vi "Get Missing Dependencies.vi"(8 "error in":errorcluster, 9 "shared directory":path, 10 "outside vis in":string[](array[string]), 11 "measurement directory":path) -> (0 "error out":errorcluster, 3 "outside vis out":string[](array[string]))   [LabVIEW 2021, in "Multiple Converter.lvlib"]
uses:
  Multiple Converter.lvlib
  e56e842d-5902-469a-bbd5-1077467e5c47.vi
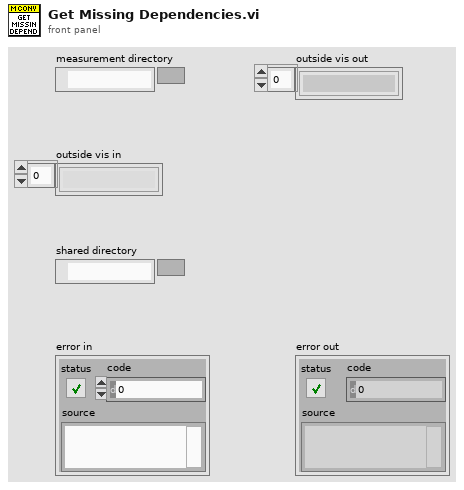
[diagram p1: front panel]
types:
  T1 = typedef "LVMissingDepInfoTypeDef.ctl" = cluster{"Missing Path":path, "Missing Name":string, "Missing Type":string}[]
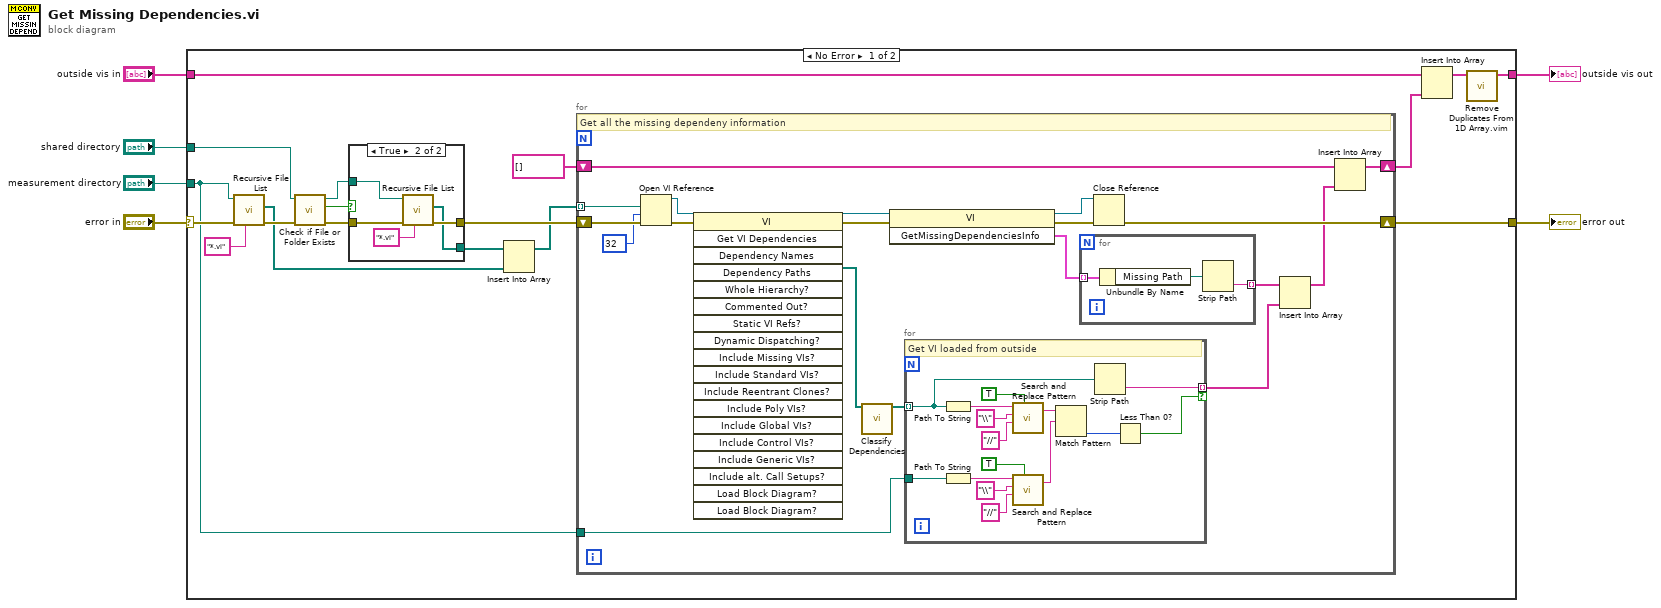
[diagram p0: block diagram]
diagram:
  n1 = case shown="No Error" "error in" {
    selector: "error in" -> [w24 w69]
    tunnel: [w21 w69] -> w5
    tunnel: "measurement directory" -> [w11 _]
    tunnel: "outside vis in" -> [w19 w68]
    tunnel: [w18 w68] -> w2
    tunnel: "shared directory" -> [w8 _]
    frame No Error {
      n2 = call <vilib>:"Recursive File List.vi"("pattern"="*.vi", "error in (no error)"=w24, "Folder Path"=w11) -> ("error out"=w16:errorcluster, "All Files in Dir"=w13:path[])  [unwired: 4 in, 3 out]
      n3 = call <vilib>:"Check if File or Folder Exists.vi"("error in (no error)"=w16, "path"=w8) -> ("error out"=w10:errorcluster, "file or folder exists?"=w9:bool, "dup path"=w7:path)  [unwired: 7 in]
      n4 = case shown="True" w9 {
        tunnel: w10 -> [w25 w29]
        tunnel: [w25 w28] -> w15
        tunnel: [_ w27] -> w14
        tunnel: w7 -> [_ w26]
        frame False {
        }
        frame True {
          n5 = call <vilib>:"Recursive File List.vi"("pattern"="*.vi", "error in (no error)"=w29, "Folder Path"=w26) -> ("error out"=w28:errorcluster, "All Files in Dir"=w27:path[])  [unwired: 4 in, 3 out]
        }
      }
      n6 = Insert Into Array(array=w14, new element=w13) -> (w12:path[])  [unwired: 1 in]
      n7 = for {
        tunnel: w12 -> [w49] mode=indexing
        shift-right: [w44] -> w21
        shift-left: w15 -> [w42]
        tunnel: w11 -> [w38]
        shift-right: [w35] -> w23
        shift-left: string[] [] -> [w36]
        # "Get all the missing dependeny information"
        n8 = Open VI Reference(vi path=w49, options=32, error in (no error)=w42) -> (vi reference=w40:refnum<vi>, error out=w48:errorcluster)  [unwired: 3 in]
        n9 = invoke class="VI" method="Get VI Dependencies"(reference=w40, error in=w48) -> (reference out=w39:refnum<vi>, error out=w41:errorcluster, "Dependency Paths"=w33:path[])  [unwired: 17 in, 16 out]
        n10 = call "Classify Dependencies.vi"("dependency paths"=w33) -> ("actual dependencies"=w32:path[])  [unwired: 13 in, 1 out]
        n11 = invoke class="VI" method="GetMissingDependenciesInfo"(reference=w39, error in=w41) -> (reference out=w43:refnum<vi>, error out=w47:errorcluster, "GetMissingDependenciesInfo"=w46:T1)  [unwired: 1 in]
        n12 = for {
          tunnel: w32 -> [w53] mode=indexing
          tunnel: w38 -> [w54]
          tunnel: [w52] -> w37 mode=indexing if=w50
          # "Get VI loaded from outside"
          n13 = Path To String(path=w53) -> (string=w61:string)
          n14 = Path To String(path=w54) -> (string=w56:string)
          n15 = call <vilib>:"Search and Replace Pattern.vi"("string"=w61, "regular expression (\"\")"="\\" ("search string"), "replace string (\"\")"="//" ("search string"), "replace all? (F)"=TRUE) -> ("result string"=w60:string)  [unwired: 1 in, 1 out]
          n16 = call <vilib>:"Search and Replace Pattern.vi"("string"=w56, "regular expression (\"\")"="\\" ("search string"), "replace string (\"\")"="//" ("search string"), "replace all? (F)"=TRUE) -> ("result string"=w55:string)  [unwired: 1 in, 1 out]
          n17 = Match Pattern(string=w60, regular expression=w55) -> (offset past match=w51:i32)  [unwired: 1 in, 3 out]
          n18 = Strip Path(path=w53) -> (name=w52:string)  [unwired: 1 out]
          n19 = Less Than 0?(x=w51) -> (x < 0?=w50:bool)
        }
        n20 = for {
          tunnel: w46 -> [w67] mode=indexing
          tunnel: [w65] -> w45 mode=indexing
          n21 = Unbundle By Name(w67) -> ("Missing Path"=w66:path)
          n22 = Strip Path(path=w66) -> (name=w65:string)  [unwired: 1 out]
        }
        n23 = Close Reference(reference=w43, error in (no error)=w47) -> (error out=w44:errorcluster)
        n24 = Insert Into Array(array=w45, new element=w37) -> (w34:string[])  [unwired: 1 in]
        n25 = Insert Into Array(array=w36, new element=w34) -> (w35:string[])  [unwired: 1 in]
      }
      n26 = Insert Into Array(array=w19, new element=w23) -> (w22:string[])  [unwired: 1 in]
      n27 = call "Remove Duplicates From 1D Array.vim"("array"=w22) -> ("array with duplicates removed"=w18:string[])  [unwired: 10 in]
    }
    frame Error {
    }
  }
  "outside vis out" <- w2
  "error out" <- w5
